vi "Read Stream and Create Channels.vi"(8 "error in (no error)":errorcluster, 10 "StreamReader Parameters in":T1, 11 "Plugin in":refnum<class "StreamReader.lvclass">) -> (0 "error out":errorcluster, 1 "Array":waveform(dbl)[](array[waveform]), 2 "StreamReader Parameters out":T1, 3 "Plugin out":refnum<class "StreamReader.lvclass">)   [LabVIEW 2024, in "StreamReader.lvlib" / "StreamReader.lvclass"]
uses:
  StreamReader.lvclass
  StreamReader Parameters.ctl
  <vilib>/FlexLogger/SDK/PluginSDK.lvlibp/PEFClasses/SDK/Producer Channel/Producer Channel.lvclass
  StreamReader Strings.vi
  <vilib>/FlexLogger/SDK/PluginSDK.lvlibp/PEFClasses/SDK/Producer Channel/Create Producer Channel.vi
  StreamReader.lvclass/StreamReader.ctl
  <vilib>/FlexLogger/SDK/PluginSDK.lvlibp
  <resource>/objmgr/ni.dex.rc
  <vilib>/FlexLogger/SDK/PluginSDK.lvlibp/PEFClasses/SDK/Plugin/Plugin.lvclass
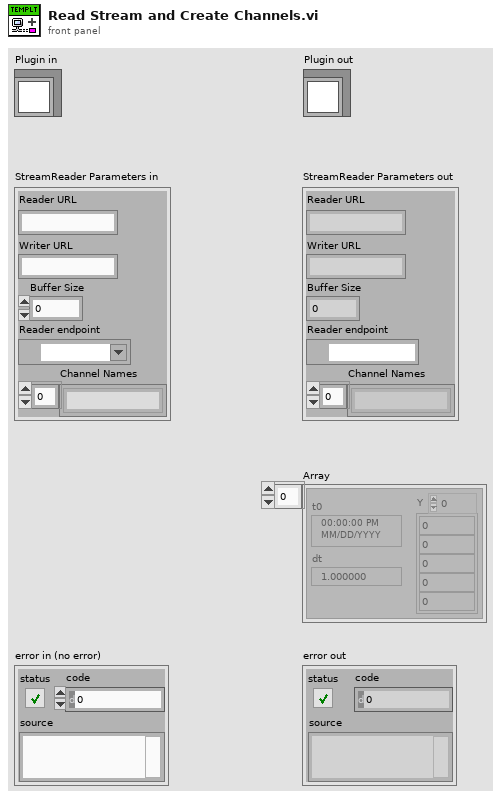
[diagram p1: front panel]
types:
  T1 = typedef "StreamReader.lvlib/StreamReader.lvclass/StreamReader Parameters.ctl" = cluster{"Reader URL":string, "Writer URL":string, "Buffer Size":i32, "Reader endpoint":refnum<k21>, "Channel Names":string[]}
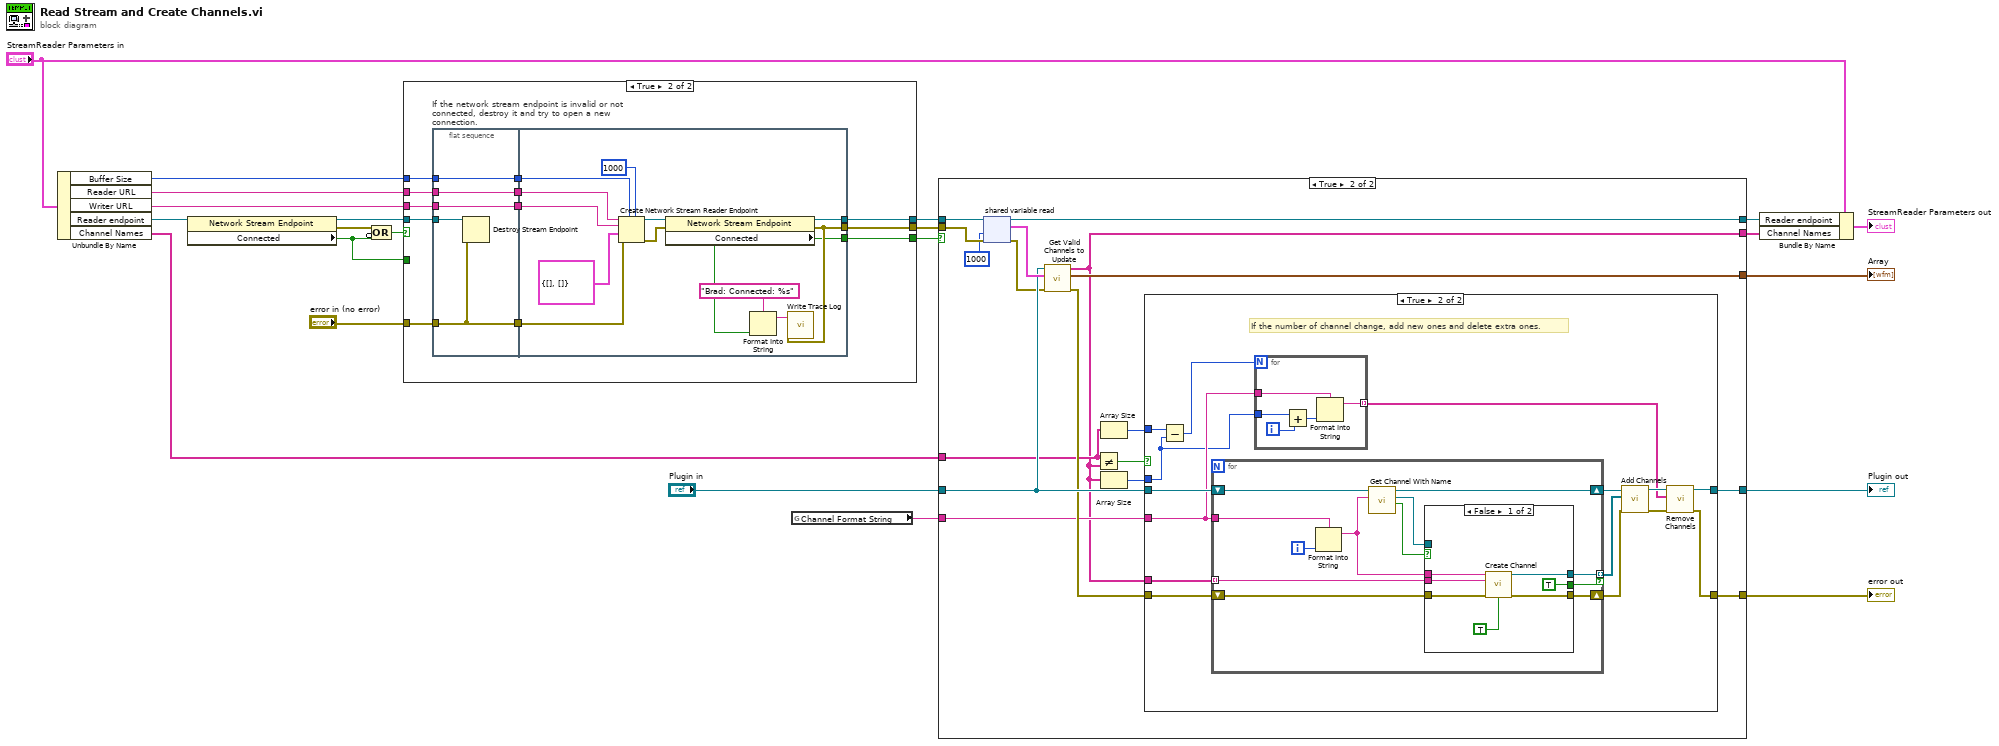
[diagram p0: block diagram]
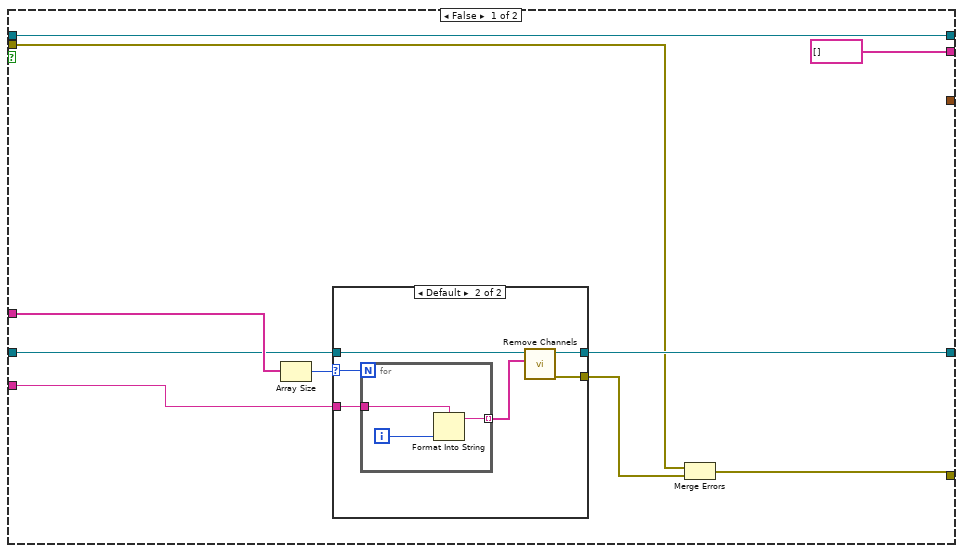
[diagram p3: hidden frame]
diagram:
  n1 = Unbundle By Name("StreamReader Parameters in") -> ("Buffer Size"=w17:i32, "Reader URL"=w18:string, "Writer URL"=w3:string, "Reader endpoint"=w16:refnum<k21>, "Channel Names"=w10:string[])
  n2 = property class="Network Stream Endpoint"(reference=w16) -> (reference out=w13:refnum<k21>, error out=w15:errorcluster, "Connected"=w12:bool)  [unwired: 1 in]
  n3 = Compound Arithmetic op=OR(w15, invert w12) -> (w14:bool)
  n4 = case shown="True" w14 {
    tunnel: [w23 w37] -> w22
    tunnel: [w25 w36] -> w21
    tunnel: [w24 w35] -> w20
    tunnel: "error in (no error)" -> [w23 w34]
    tunnel: w18 -> [_ w33]
    tunnel: w17 -> [_ w32]
    tunnel: w13 -> [w24 w28]
    tunnel: w12 -> [w25 _]
    tunnel: w3 -> [_ w27]
    frame False {
    }
    frame True {
      n5 = flat-sequence "If the network stream endpoint is invalid or not connected, destroy it and try to open a new connection." {
        tunnel: w32 -> [w41]
        tunnel: w33 -> [w42]
        tunnel: w34 -> [w39]
        tunnel: [w39] -> w31
        tunnel: [w42] -> w30
        tunnel: [w41] -> w29
        tunnel: w28 -> [w40]
        tunnel: w27 -> [w38]
        tunnel: [w38] -> w26
        tunnel: [w46] -> w37
        tunnel: [w43] -> w36
        tunnel: [w52] -> w35
        tunnel: w31 -> [w51]
        tunnel: w30 -> [w48]
        tunnel: w29 -> [w50]
        tunnel: w26 -> [w49]
        frame #0 {
          n6 = Destroy Stream Endpoint(8:w39, 11:w40) -> ()  [unwired: 1 out]
        }
        frame #1 {
          n7 = Create Network Stream Reader Endpoint(5:1000 ("timeout in ms (-1)"), 7:w50, 8:w51, 9:cluster{waveform(dbl)[], string[]} {[], []}, 10:w49, 11:w48) -> (0:w54:errorcluster, 3:w55:refnum<k21>)  [unwired: 1 in]
          n8 = property class="Network Stream Endpoint"(reference=w55, error in=w54) -> (reference out=w52:refnum<k21>, error out=w46:errorcluster, "Connected"=w43:bool)
          n9 = Format Into String(format string="Brad: Connected: %s", w43) -> (resulting string=w45:string)  [unwired: 2 in, 1 out]
          n10 = call <vilib>:"Write Trace Log.vi"("error in (no error)"=w46, "Message"=w45) -> ()  [unwired: 9 in, 1 out]
        }
      }
    }
  }
  n11 = global read "StreamReader Strings.vi" "Channel Format String"() -> (w1:string)
  n12 = case shown="True" w21 {
    tunnel: w20 -> [w65 w92]
    tunnel: w22 -> [w57 w91]
    tunnel: [w56 w89] -> w8
    tunnel: [w65 w87] -> w6
    tunnel: "Plugin in" -> [w61 w85]
    tunnel: [w60 w90] -> w11
    tunnel: w10 -> [w63 w79]
    tunnel: [_ w88] -> w9
    tunnel: [string[] [] ("Channels Out") w78] -> w5
    tunnel: w1 -> [w64 w81]
    frame False {
      n13 = Array Size(array=w63) -> (size(s)=w59:i32)
      n14 = case shown="Default" w59 {
        selector: w59 -> [_ w67]
        tunnel: w64 -> [_ w71]
        tunnel: w61 -> [w66 w70]
        tunnel: [_ w69] -> w58
        tunnel: [w66 w68] -> w60
        frame 0 {
        }
        frame Default {
          n15 = for {
            N: w67 -> [_]
            tunnel: [w75] -> w72 mode=indexing
            tunnel: w71 -> [w74]
            i -> [w73]
            n16 = Format Into String(format string=w74, w73) -> (resulting string=w75:string)  [unwired: 2 in, 1 out]
          }
          n17 = call-dynamic "Remove Channels.vi"("Unique Channel Identifiers to Delete"=w72, "Plugin in"=w70) -> ("error out"=w69:errorcluster, "Plugin out"=w68:refnum<class "StreamReader.lvclass">)  [unwired: 8 in]
        }
      }
      n18 = Merge Errors(w57, w58) -> (w56:errorcluster)
    }
    frame True {
      n19 = shared-variable-read(w92, w91, 1000 ("timeout ms (-1)")) -> (w87:refnum<k21>, w84:errorcluster, w86:cluster{waveform(dbl)[], string[]})  [unwired: 1 out]
      n20 = call "Get Valid Channels to Update.vi"("error in (no error)"=w84, "Data Read"=w86, "Plugin in"=w85) -> ("error out"=w83:errorcluster, "Waveforms Out"=w88:waveform(dbl)[], "Channels Out"=w78:string[])  [unwired: 6 in]
      n21 = Not Equal?(x=w79, y=w78) -> (x != y?=w82:bool)
      n22 = Array Size(array=w79) -> (size(s)=w76:i32)
      n23 = Array Size(array=w78) -> (size(s)=w77:i32)
      n24 = case shown="True" w82 {
        tunnel: w83 -> [w94 w109]
        tunnel: [w94 w95] -> w89
        tunnel: w85 -> [w93 w108]
        tunnel: w78 -> [_ w107]
        tunnel: [w93 w97] -> w90
        tunnel: w81 -> [_ w104]
        tunnel: w77 -> [_ w103]
        tunnel: w76 -> [_ w106]
        frame False {
        }
        frame True {
          # "If the number of channel change, add new ones and delete extra ones."
          n25 = Subtract(x=w106, y=w103) -> (x-y=w105:i32)
          n26 = for {
            tunnel: w107 -> [w116] mode=indexing
            shift-right: [w125] -> w98
            shift-left: w109 -> [w126]
            tunnel: [w124] -> w99 mode=indexing if=w115
            shift-right: [w120] -> w100
            shift-left: w108 -> [w121]
            tunnel: w104 -> [w118]
            i -> [w122]
            n27 = Format Into String(format string=w118, w122) -> (resulting string=w119:string)  [unwired: 2 in, 1 out]
            n28 = call <vilib>:"Get Channel With Name.vi"("Name"=w119, "Plugin in"=w121) -> ("Found?"=w123:bool, "Channel"=w117:refnum<class "Channel.lvclass">, "Plugin out"=w120:refnum<class "StreamReader.lvclass">)  [unwired: 7 in]
            n29 = case shown="False" w123 {
              tunnel: w126 -> [w133 w134]
              tunnel: [w131 w134] -> w125
              tunnel: [w132 _] -> w124
              tunnel: w116 -> [w129 _]
              tunnel: w119 -> [w130 _]
              tunnel: w117 -> [_ _]
              tunnel: [TRUE _] -> w115
              frame False {
                n30 = call-poly <vilib>:"Create Channel.vi"("Unique Channel Identifier"=w130, "Default Channel Name"=w129, "error in (no error)"=w133, "Can Disable?"=TRUE) -> ("Producer Channel"=w132:refnum<class "Producer Channel.lvclass">, "error out"=w131:errorcluster)  [unwired: 10 in]
              }
              frame True {
              }
            }
          }
          n31 = for {
            N: w105 -> [_]
            tunnel: w103 -> [w114]
            tunnel: [w111] -> w96 mode=indexing
            tunnel: w104 -> [w110]
            i -> [w113]
            n32 = Add(x=w114, y=w113) -> (x+y=w112:i32)
            n33 = Format Into String(format string=w110, w112) -> (resulting string=w111:string)  [unwired: 2 in, 1 out]
          }
          n34 = call <vilib>:"Add Channels.vi"("error in (no error)"=w98, "Channels"=w99, "Plugin in"=w100) -> ("error out"=w102:errorcluster, "Plugin out"=w101:refnum<class "StreamReader.lvclass">)  [unwired: 7 in]
          n35 = call-dynamic "Remove Channels.vi"("error in (no error)"=w102, "Unique Channel Identifiers to Delete"=w96, "Plugin in"=w101) -> ("error out"=w95:errorcluster, "Plugin out"=w97:refnum<class "StreamReader.lvclass">)  [unwired: 7 in]
        }
      }
    }
  }
  "error out" <- w8
  "Plugin out" <- w11
  "Array" <- w9
  n36 = Bundle By Name(cluster="StreamReader Parameters in", "Reader endpoint"=w6, "Channel Names"=w5) -> (→"StreamReader Parameters out":T1)
